vi "PingPong.2BitCounter.vi"(7 "Increment":bool, 13 "Reset":bool) -> (8 "Counter Value":fxp<+,2,2>)   [LabVIEW 2014]
panel:
  # "Copyright 2014 Vidrio Technologies\nScanImage 5 software is licensed under the Apache License, Version 2.0 (the \"License\"); you may not use any files contained\nwithin the ScanImage 5 release except in compliance with the License. You may obtain a copy of the License at\n http://www.apache.org/licenses/LICENSE-2.0\nUnless required by applicable law or agreed to in writing, software distributed under the License is distributed on an\n\"AS IS\" BASIS, WITHOUT WARRANTIES OR CONDITIONS OF ANY KIND, either express or implied. See the License for the\n specific language governing permissions and limitations under the License."
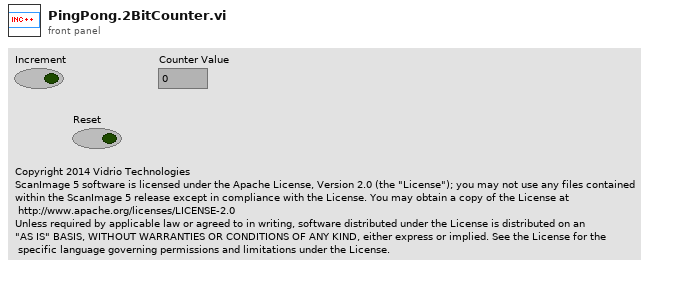
[diagram p1: front panel]
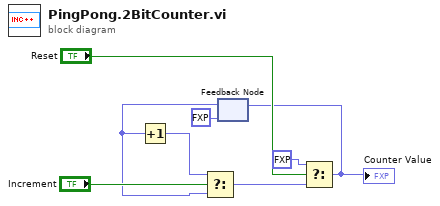
[diagram p0: block diagram]
diagram:
  n1 = feedback #1(fxp<+,2,2> 0.0) -> (w5:fxp<+,2,2>)
  n2 = Increment(x=w5) -> (x+1=w7:fxp<+,2,2>)
  n3 = Select(t=w7, s="Increment", f=w5) -> (s? t:f=w4:fxp<+,2,2>)
  n4 = Select(t=fxp<+,2,2> 0.0, s="Reset", f=w4) -> (s? t:f=w1:fxp<+,2,2>)
  "Counter Value" <- w1
  n5 = feedback-in #1(w1) -> ()
